vi "Read AO.vi"(0 "FPGA API in":refnum<class "FPGA API Concrete.lvclass">, 11 "error in (no error)":errorcluster) -> (4 "FPGA API out":refnum<class "FPGA API Concrete.lvclass">, 6 "AO":dbl[](array[numeric]), 15 "error out":errorcluster)   [LabVIEW 2019, in "FPGA API Concrete.lvclass"]
uses:
  FPGA API Concrete.lvclass
  FPGA API Concrete.lvclass/FPGA API Concrete.ctl
  <vilib>/Utility/error.llb/Error Cluster From Error Code.vi
  <vilib>/rvi/errors/niLvFpgaAdjustHostInterfaceError.vi
  <vilib>/rvi/interface/nirviReadWriteControl/nirviReadWriteControl.xnode
  FPGA Ref.ctl
  NiFpgaLv.dll
  <vilib>/rvi/interface/Simulation/niFpgaSimulationCallBeginRW.vi
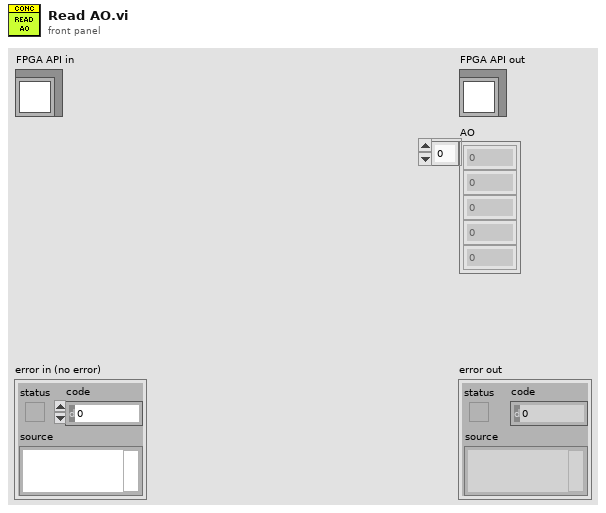
[diagram p1: front panel]
types:
  T1 = typedef "FPGA API Concrete.lvclass/FPGA Ref.ctl" = refnum<k20>
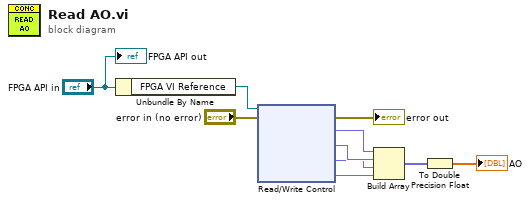
[diagram p0: block diagram]
diagram:
  n1 = Unbundle By Name("FPGA API in") -> ("FPGA VI Reference"=w9:T1)
  n2 = xnode "Read/Write Control"("FPGA VI Reference In"=w9, "error in"="error in (no error)") -> ("error out"=→"error out":errorcluster, "Mod5/AO0"=w6:fxp<+/-,20,5>, "Mod5/AO1"=w5:fxp<+/-,20,5>, "Mod5/AO2"=w4:fxp<+/-,20,5>, "Mod5/AO3"=w3:fxp<+/-,20,5>)  [unwired: 1 out]
  n3 = Build Array(w6, w5, w4, w3) -> (w2:fxp<+/-,20,5>[])
  n4 = To Double Precision Float(number=w2) -> (double precision float=→"AO":dbl[])
  "FPGA API out" <- "FPGA API in"
